vi "FT_Open_Device_By_Serial_Number.vi"(0 "Device Serial Number":string) -> (1 "FT_Status":u32(ring) items=["FT_OK", "FT_INVALID_HANDLE", "FT_DEVICE_NOT_FOUND", "FT_DEVICE_NOT_OPENED", "FT_IO_ERROR", "FT_INSUFFICIENT_RESOURCES", "FT_INVALID_PARAMETER", "FT_INVALID_BAUD_RATE", "FT_DEVICE_NOT_OPENED_FOR_ERASE", "FT_DEVICE_NOT_OPENED_FOR_WRITE", "FT_FAILED_TO_WRITE_DEVICE", "FT_EEPROM_READ_FAILED", "FT_EEPROM_WRITE_FAILED", "FT_EEPROM_ERASE_FAILED", "FT_EEPROM_NOT_PRESENT", "FT_EEPROM_NOT_PROGRAMMED", "FT_INVALID_ARGS", "FT_NOT_SUPPORTED", "FT_OTHER_ERROR"], 2 "Handle":u64)   [LabVIEW 2018]
uses:
  FTD2XX.dll
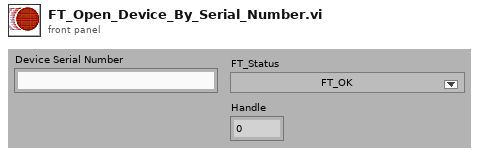
[diagram p1: front panel]
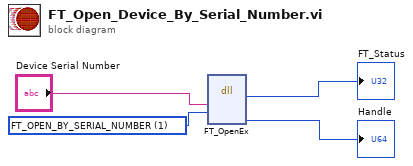
[diagram p0: block diagram]
diagram:
  w1 = u32 1 items=["FT_OPEN_BY_SERIAL_NUMBER"=1, "FT_OPEN_BY_DESCRIPTION"=2, "FT_OPEN_BY_LOCATION"=4] ("Flags")
  n1 = dll-call lib="FTD2XX.dll" fn="FT_OpenEx"("SerialNumber"="Device Serial Number", "Flags"=w1) -> ("FT_Status"=→"FT_Status":u32, "Handle"=→"Handle":u64)  [unwired: 6 in, 2 out]
